vi "OSC_config_UI.vi"() -> ()   [LabVIEW 2012]
uses:
  SubVIs/controls/scale.ctl
  SubVIs/controls/sampling_rate.ctl
  global.vi
  <vilib>/Platform/browser.llb/Open URL in Default Browser (string).vi
  libaries/Tektronix 7000 Series/Tektronix 7000 Series.lvlib
panel:
  in  "Help Button":bool
  out "Fast Frame count":i32=2
  in  "RESET?":bool
  in  "configure":bool
  out "resolution (Hz)":ext=24999.999999999999998 format="%#_6p"
  out "sampling interval (s)":ext=2e-10 format="%#_6p"
  out "waveform length (s)":ext=0.000040000000000000000003 format="%#_6p"
  in  "horizontal scale (t/div)":T1=4e-06 items=["400ns/div"=4e-07, "1µs/div"=1e-06, "2µs/div"=2e-06, "4µs/div"=4e-06, "10µs/div"=1e-05, "20µs/div"=2e-05]
  in  "sampling rate (Hz)":T2=5000000000.0 items=["20 GHz (50ps/sample)", "10 GHz (100ps/sample)", "5.0 GHz (200ps/sample)", "2.5 GHz (400ps/sample)", "1.25 GHz (0.8ns/sample)", "0.5 GHz (2ns/sample)"]
  out "sample points":i32=200000
  in  "Close":bool
  # "Configure Oscilloscope"
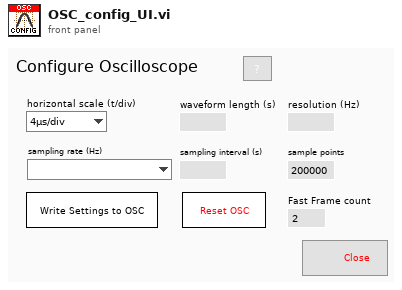
[diagram p1: front panel]
types:
  T1 = typedef "scale.ctl" = dbl
  T2 = typedef "sampling_rate.ctl" = ext
  T3 = enum16{"load busy", "unload busy", "show busy", "hide busy"}
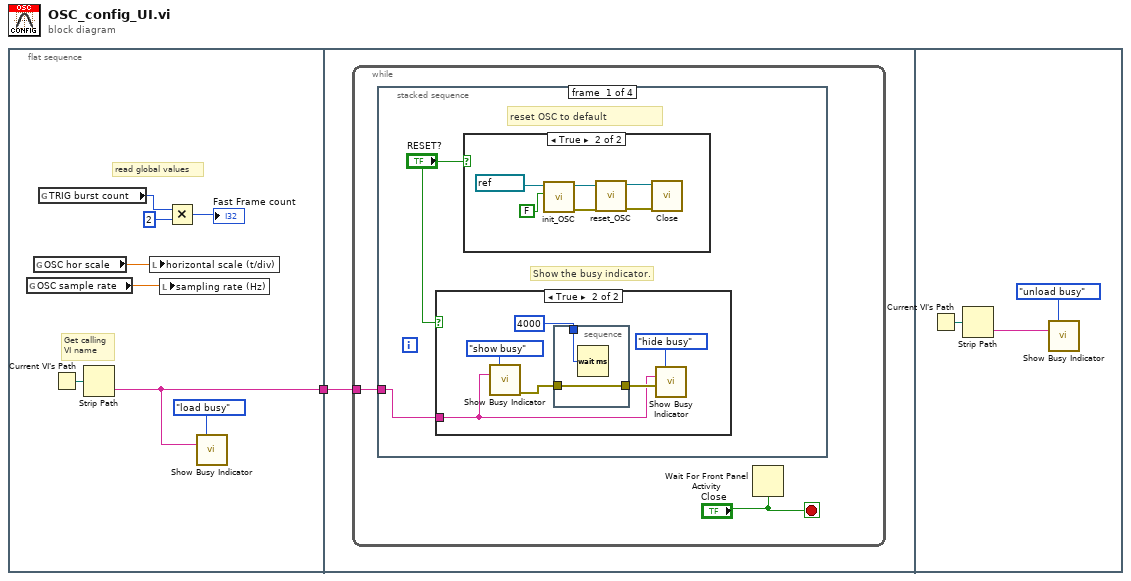
[diagram p0: block diagram]
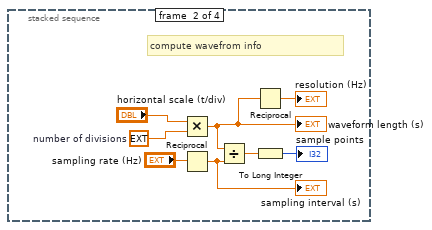
[diagram p4: hidden frame]
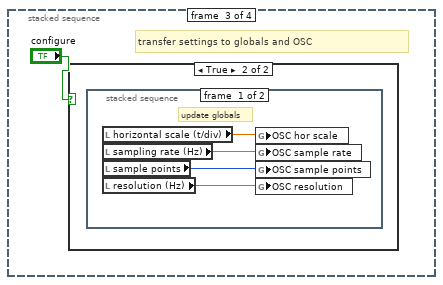
[diagram p5: hidden frame]
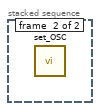
[diagram p7: hidden frame]
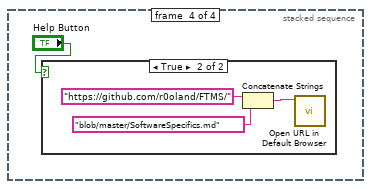
[diagram p8: hidden frame]
diagram:
  n1 = flat-sequence {
    tunnel: [w5] -> w1
    tunnel: w1 -> [w10]
    frame #0 {
      # "Get calling\nVI name"
      # "read global values"
      n2 = global read "global.vi" "OSC sample rate"() -> (w8:T2)
      n3 = global read "global.vi" "OSC hor scale"() -> (w9:T1)
      n4 = global read "global.vi" "TRIG burst count"() -> (w3:i32)
      n5 = Current VI's Path() -> (path=w7:path)
      n6 = Strip Path(path=w7) -> (name=w5:string)  [unwired: 1 out]
      n7 = local write "horizontal scale (t/div)"(w9) -> ()
      n8 = local write "sampling rate (Hz)"(w8) -> ()
      n9 = Multiply(x=w3, y=2) -> (x*y=→"Fast Frame count":i32)
      n10 = call "Show Busy Indicator.vi"("Command"=T3."load busy", "Calling VI Name"=w5) -> ()  [unwired: 13 in, 1 out]
    }
    frame #1 {
      n11 = while {
        tunnel: w10 -> [w11]
        stop <- "Close" stop-if-true
        n12 = stacked-sequence {
          tunnel: w11 -> [w13 _ _ _]
          frame #0 {
            # "Show the busy indicator."
            # "reset OSC to default"
            n13 = case shown="True" "RESET?" {
              tunnel: w13 -> [_ w15]
              frame False {
              }
              frame True {
                n14 = call "Show Busy Indicator.vi"("Command"=T3."show busy", "Calling VI Name"=w15) -> ("error out"=w18:errorcluster)  [unwired: 13 in]
                n15 = stacked-sequence {
                  tunnel: w18 -> [w22]
                  tunnel: [w22] -> w17
                  tunnel: u32 4000 ("milliseconds to wait") -> [w21]
                  frame #0 {
                    n16 = Wait (ms)(milliseconds to wait=w21) -> ()  [unwired: 1 out]
                  }
                }
                n17 = call "Show Busy Indicator.vi"("Command"=T3."hide busy", "Calling VI Name"=w15, "error in (no error)"=w17) -> ()  [unwired: 12 in, 1 out]
              }
            }
            n18 = case shown="True" "RESET?" {
              frame False {
              }
              frame True {
                n19 = call "init_OSC.vi"("reset (f)"=FALSE, "VISA resource name"=refnum<visa-resource-name> "OSC" ("OSC")) -> ("error out"=w25:errorcluster, "VISA resource name out"=w26:refnum<visa-resource-name>)  [unwired: 8 in]
                n20 = call "reset_OSC.vi"("error in (no error)"=w25, "VISA resource name"=w26) -> ("error out"=w23:errorcluster, "VISA resource name out"=w24:refnum<visa-resource-name>)  [unwired: 8 in]
                n21 = call "Close.vi"("error in (no error)"=w23, "VISA resource name"=w24) -> ()  [unwired: 9 in, 1 out]
              }
            }
          }
          frame #1 {
            w36 = ext 10.0  # number of divisions
            # "compute wavefrom info"
            n22 = Multiply(x="horizontal scale (t/div)", y=w36) -> (x*y=w30:ext)
            "waveform length (s)" <- w30
            n23 = Reciprocal(x="sampling rate (Hz)") -> (1/x=w33:T2)
            "sampling interval (s)" <- w33
            n24 = Divide(x=w30, y=w33) -> (x/y=w32:T2)
            n25 = Reciprocal(x=w30) -> (1/x=→"resolution (Hz)":ext)
            n26 = To Long Integer(number=w32) -> (32bit integer=→"sample points":i32)
          }
          frame #2 {
            # "transfer settings to globals and OSC"
            n27 = case shown="True" "configure" {
              frame False {
              }
              frame True {
                n28 = stacked-sequence {
                  frame #0 {
                    # "update globals"
                    n29 = local read "horizontal scale (t/div)"() -> (w41:T1)
                    n30 = local read "sampling rate (Hz)"() -> (w40:T2)
                    n31 = local read "sample points"() -> (w39:i32)
                    n32 = local read "resolution (Hz)"() -> (w38:ext)
                    n33 = global write "global.vi" "OSC hor scale"(w41) -> ()
                    n34 = global write "global.vi" "OSC sample rate"(w40) -> ()
                    n35 = global write "global.vi" "OSC sample points"(w39) -> ()
                    n36 = global write "global.vi" "OSC resolution"(w38) -> ()
                  }
                  frame #1 {
                    n37 = call "set_OSC.vi"() -> ()  [unwired: 12 in]
                  }
                }
              }
            }
          }
          frame #3 {
            n38 = case shown="True" "Help Button" {
              frame False {
              }
              frame True {
                n39 = Concatenate Strings("https://github.com/r0oland/FTMS/" ("string"), "blob/master/SoftwareSpecifics.md" ("string")) -> (w43:string)
                n40 = call-poly <vilib>:"Open URL in Default Browser.vi"("URL"=w43) -> ()  [unwired: 5 in, 2 out]
              }
            }
          }
        }
        n41 = Wait For Front Panel Activity(3:"Close") -> ()  [unwired: 2 in, 1 out]
      }
    }
    frame #2 {
      n42 = Current VI's Path() -> (path=w47:path)
      n43 = Strip Path(path=w47) -> (name=w46:string)  [unwired: 1 out]
      n44 = call "Show Busy Indicator.vi"("Command"=T3."unload busy", "Calling VI Name"=w46) -> ()  [unwired: 13 in, 1 out]
    }
  }
